vi "Statistics.vi"(10 "data":u16[][](array[numeric])) -> (2 "Average":dbl, 3 "StDev":dbl)   [LabVIEW 2014]
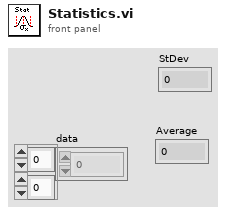
[diagram p1: front panel]
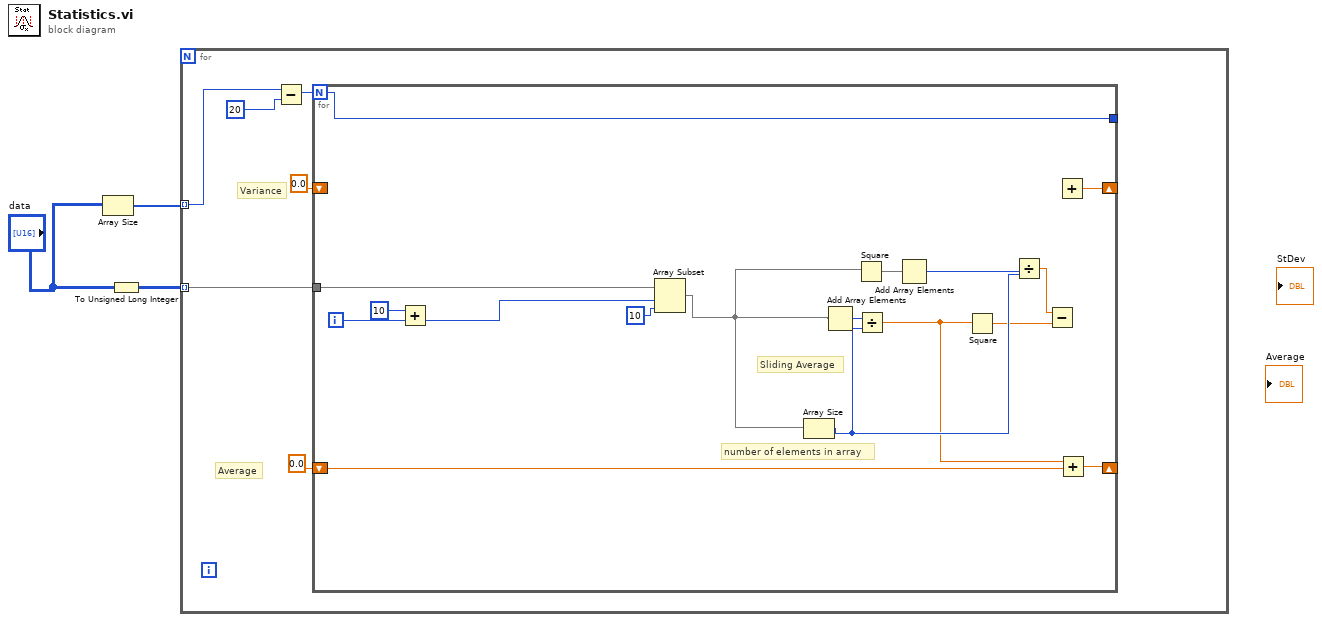
[diagram p0: block diagram]
diagram:
  n1 = Array Size(array="data") -> (size(s)=w1:i32[])
  n2 = To Unsigned Long Integer(number="data") -> (unsigned 32bit integer=w3:u32[][])
  n3 = for {
    tunnel: w3 -> [w9] mode=indexing
    tunnel: w1 -> [w8] mode=indexing
    # "Variance"
    # "Average"
    n4 = Subtract(x=w8, y=20) -> (x-y=w7:i32)
    n5 = for {
      N: w7 -> [w12]
      tunnel: w9 -> [w26]
      shift-right: [w14] -> _
      shift-left: 0.0 ("x") -> [w10]
      shift-right: [w13] -> _
      shift-left: 0.0 ("x") -> [_]
      tunnel: [w12] -> _
      i -> [w23]
      # "number of elements in array"
      # "Sliding Average"
      n6 = Add(x=10, y=w23) -> (x+y=w22:i32)
      n7 = Array Subset(array=w26, index=w22, length=10) -> (w18:u32[])
      n8 = Array Size(array=w18) -> (size(s)=w19:i32)
      n9 = Add Array Elements(numeric array=w18) -> (sum=w25:u32)
      n10 = Square(x=w18) -> (x^2=w24:u32[])
      n11 = Divide(x=w25, y=w19) -> (x/y=w11:dbl)
      n12 = Add Array Elements(numeric array=w24) -> (sum=w17:u32)
      n13 = Square(x=w11) -> (x^2=w15:dbl)
      n14 = Divide(x=w17, y=w19) -> (x/y=w16:dbl)
      n15 = Subtract(x=w16, y=w15) -> ()  [unwired: 1 out]
      n16 = Add() -> (x+y=w13:dbl)  [unwired: 2 in]
      n17 = Add(x=w11, y=w10) -> (x+y=w14:dbl)
    }
  }
